vi "Read SessionState.vi"(8 "error in (no error)":errorcluster, 11 "Session in":refnum<class "Session.lvclass">) -> (0 "error out":errorcluster, 2 "Session State":T1, 3 "Session out":refnum<class "Session.lvclass">)   [LabVIEW 2013, in "MQTT Server.lvlib" / "Session.lvclass"]
uses:
  Session.lvclass
  Session State -- cluster.ctl
  Control Packets/SUBSCRIBE/Topic Subscription -- cluster.ctl
  Control Packets/ControlPacket/QualityOfService -- enum.ctl
  Control Packets/ControlPacket/Pending Transmission -- cluster.ctl
  Control Packets/ControlPacket/ControlPacket.lvclass
  Session.lvclass/Session.ctl
  Control Packets/SUBSCRIBE/SUBSCRIBE.lvclass
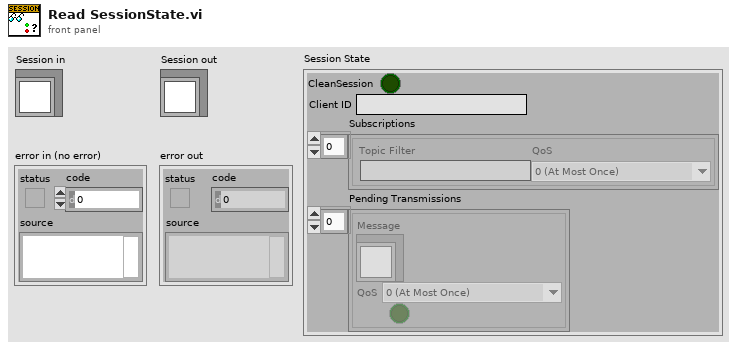
[diagram p1: front panel]
types:
  T1 = typedef "MQTT Server.lvlib/Session.lvclass/Session State -- cluster.ctl" = cluster{"CleanSession":bool, "Client ID":string, "Subscriptions":T2[], "Pending Transmissions":T4[]}
  T2 = typedef "SUBSCRIBE.lvclass/Topic Subscription -- cluster.ctl" = cluster{"Topic Filter":string, "QoS":T3}
  T3 = typedef "ControlPacket.lvclass/QualityOfService -- enum.ctl" = enum16{"0 (At Most Once)", "1 (At Least Once)", "2 (Exactly Once)"}
  T4 = typedef "ControlPacket.lvclass/Pending Transmission -- cluster.ctl" = cluster{"Message":refnum<class "ControlPacket.lvclass">, "QoS":T3, "Tx-Rx":bool}
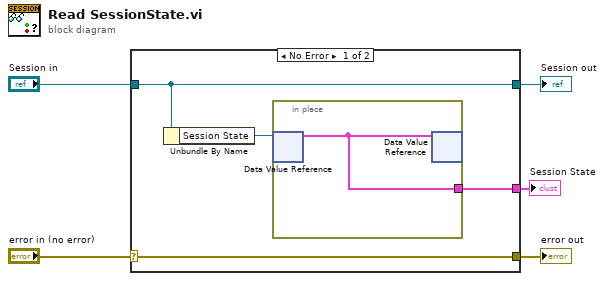
[diagram p0: block diagram]
diagram:
  n1 = case shown="No Error" "error in (no error)" {
    selector: "error in (no error)" -> [w9 w11]
    tunnel: [w9 w11] -> w4
    tunnel: [w7 w12] -> w2
    tunnel: "Session in" -> [w7 w12]
    tunnel: [w6 _] -> w1
    frame No Error {
      n2 = Unbundle By Name(w7) -> ("Session State"=w8:refnum<data-value>)
      n3 = in-place {
        in-place-border: [w10] -> w6
        n4 = in-place-dvr #1(w8) -> (w10:T1)  [unwired: 1 out]
        n5 = in-place-dvr #1(w10) -> ()  [unwired: 2 out]
      }
    }
    frame Error {
    }
  }
  "error out" <- w4
  "Session out" <- w2
  "Session State" <- w1
